vi "codigo 3.vi"() -> ()   [LabVIEW 2019]
panel:
  out "Intensity Graph":dbl[][](graph)
  in  "Array":dbl[](array[knob]) scale=0.0..10.0
  in  "Ring":u16(ring)
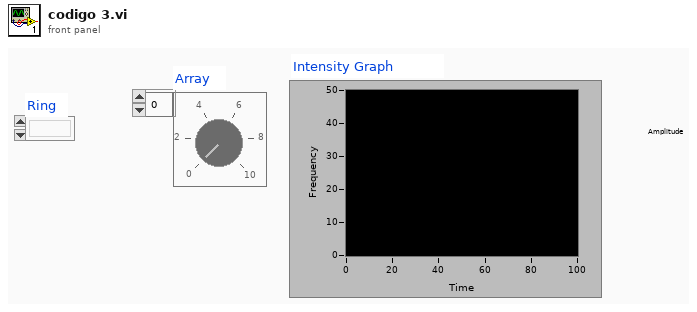
[diagram p1: front panel]
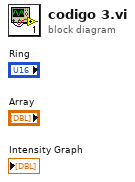
[diagram p0: block diagram]
diagram:
